vi "TestExec.Test Metric Add_Get.vi"(7 "Log Dir":path=path "C:/MTE/Circle Test/Logs", 8 "Max Hist Len":i32=10000, 9 "Test Record":T2, 10 "Action":T1, 11 "Test Result Metrics":T5) -> (1 "Test History":T4, 3 "Test Result Metrics Out":T5)   [LabVIEW 2018]
uses:
  TestExec.Test Result Metric Status.ctl
  TestExec.Test Result Metric History.ctl
  TestExec.Test Result Metric History Item.ctl
  <vilib>/KATE/SeqMgr/SeqMgr.Result State Enum.ctl
  TestExec.Test Metric Action Selector.ctl
  <vilib>/KATE/Files/File Utils.lvlib
  <vilib>/KATE/SeqMgr/SeqMgr.lvlib
panel:
  # "Time                                           Test/UUT                      Result/Code                                 Description"
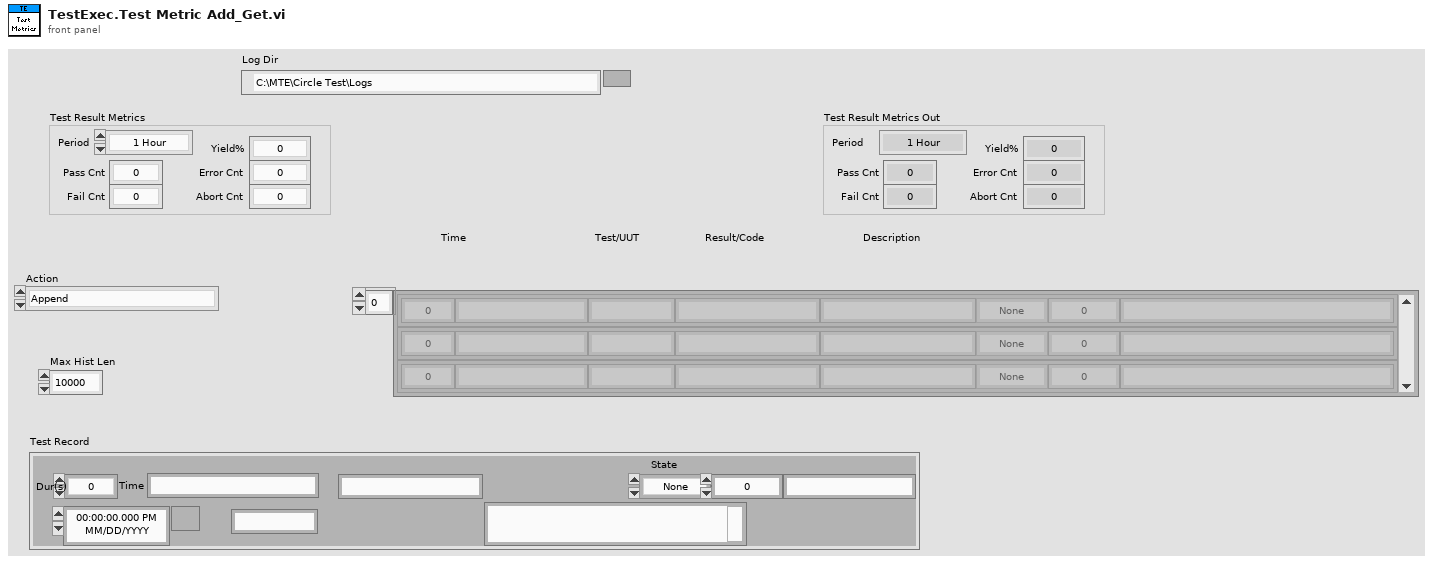
[diagram p1: front panel]
types:
  T1 = typedef "TestExec.Test Metric Action Selector.ctl" = enum16{"Append", "Get Metrics", "Reset", "Load", "Save"}
  T2 = typedef "TestExec.Test Result Metric History Item.ctl" = cluster{"TimeStamp":timestamp, "Dur(s)":dbl, "Time":string, "Mode ":string, "Test ":string, "SN":string, "State":T3, "Code":i32, "Description":string}
  T3 = typedef "KATE_Lib.lvlib/SeqMgr.lvlib/SeqMgr.Result State Enum.ctl" = enum16{"None", "Passing", "Failing", "PASS", "FAIL", "ABORT", "ERROR"}
  T4 = typedef "TestExec.Test Result Metric History.ctl" = T2[]
  T5 = typedef "TestExec.Test Result Metric Status.ctl" = cluster{"Period":enum16{"1 Hour", "4 Hours", "1 Day", "1 Week"}, "Pass Cnt":i32, "Fail Cnt":i32, "Yield%":dbl, "Error Cnt":i32, "Abort Cnt":i32}
  T6 = enum16{"open", "replace", "create", "open or create", "replace or create", "replace or create with confirmation"}
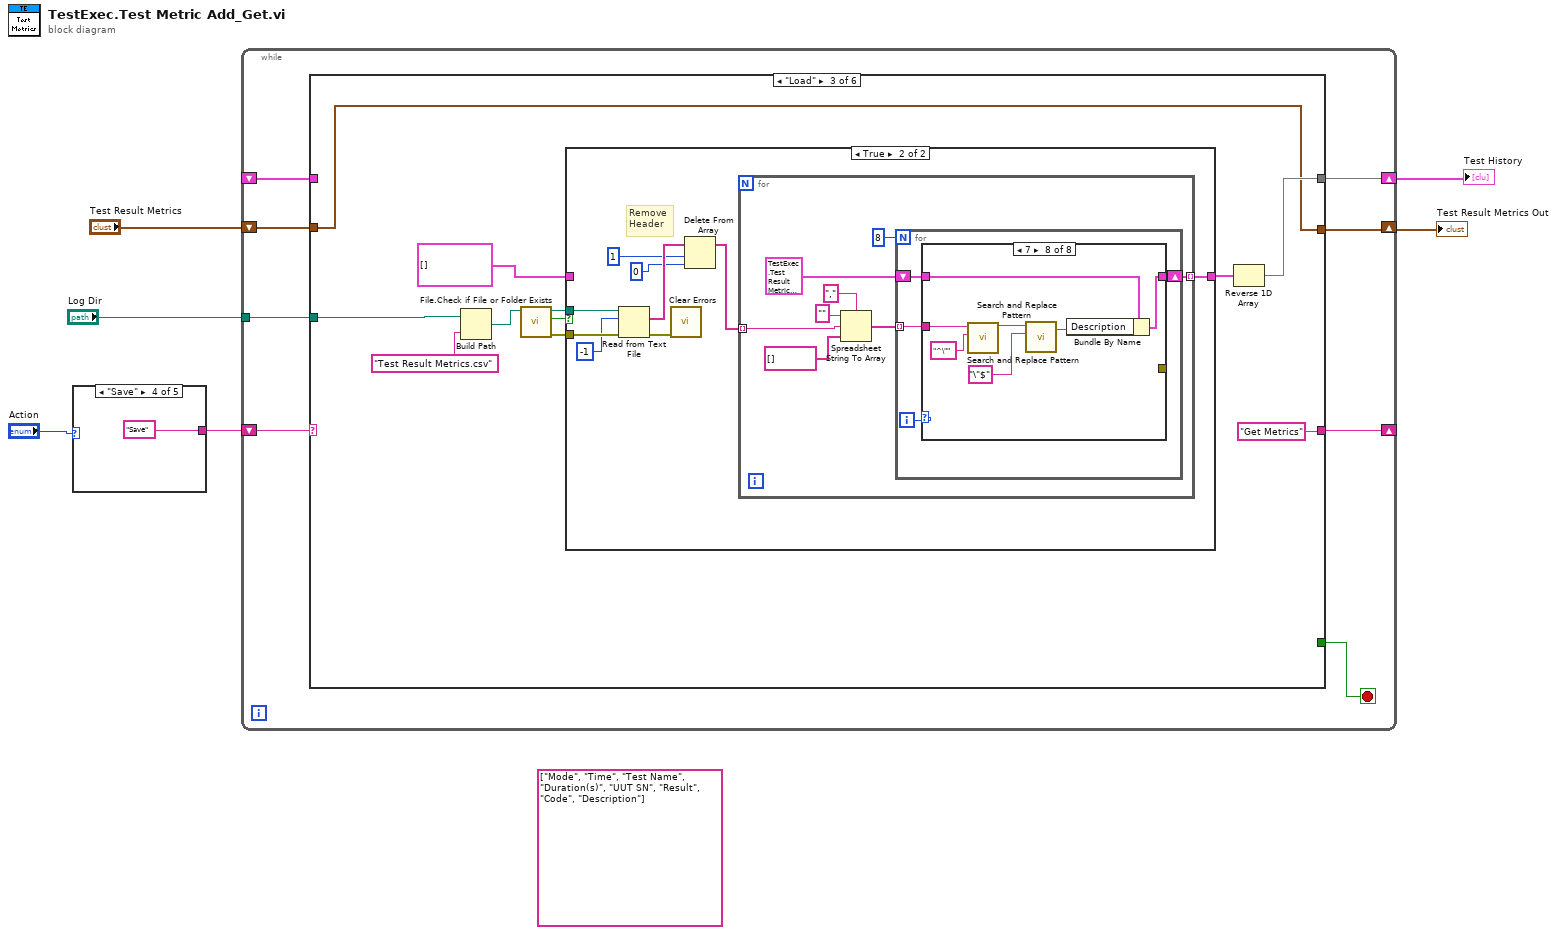
[diagram p0: block diagram]
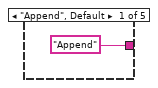
[diagram p2: hidden frame]
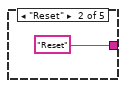
[diagram p3: hidden frame]
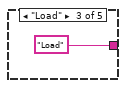
[diagram p4: hidden frame]
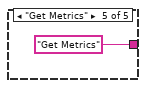
[diagram p5: hidden frame]
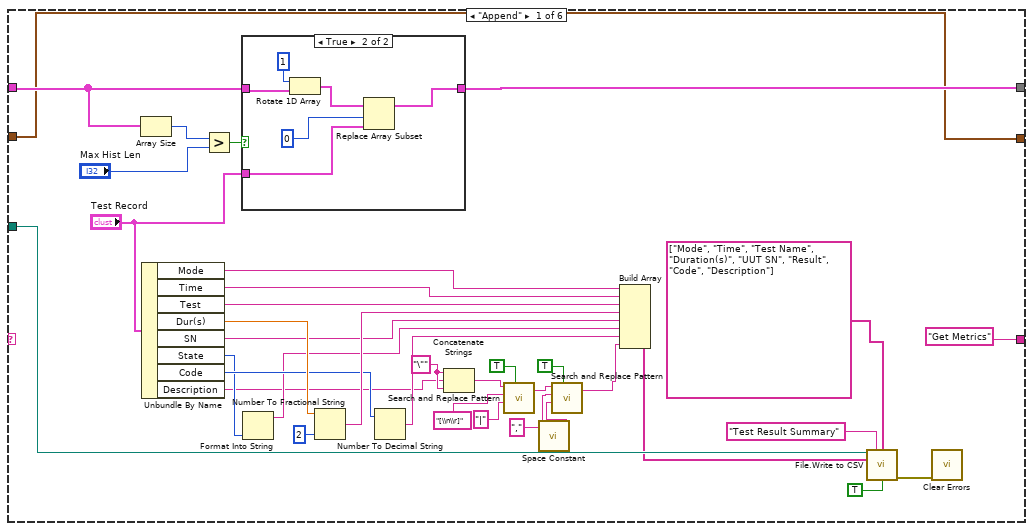
[diagram p6: hidden frame]
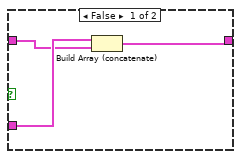
[diagram p7: hidden frame]
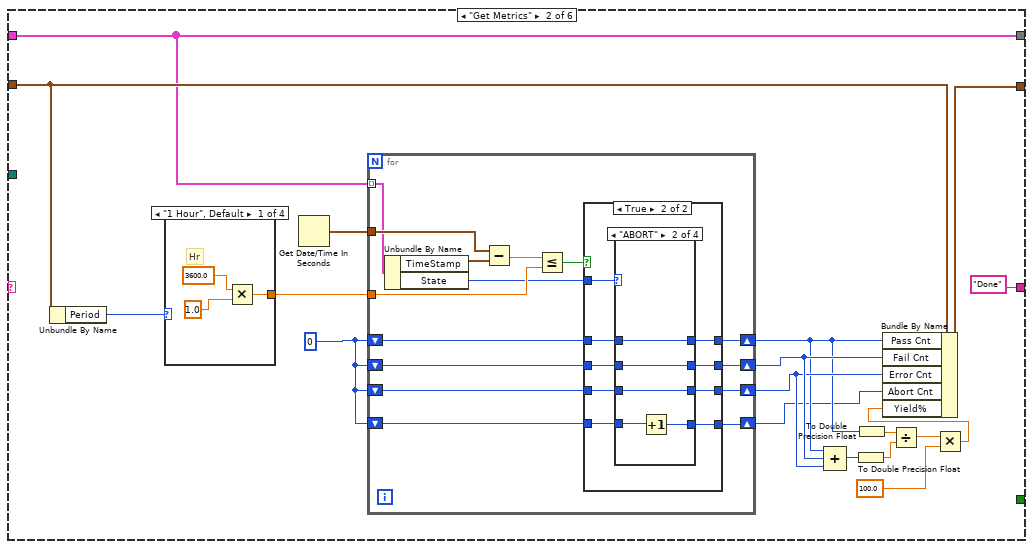
[diagram p8: hidden frame]
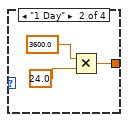
[diagram p9: hidden frame]
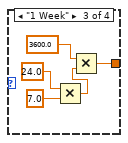
[diagram p10: hidden frame]
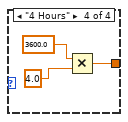
[diagram p11: hidden frame]
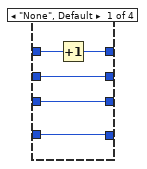
[diagram p13: hidden frame]
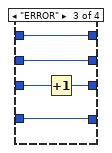
[diagram p14: hidden frame]
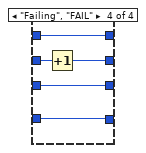
[diagram p15: hidden frame]
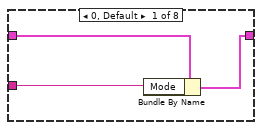
[diagram p17: hidden frame]
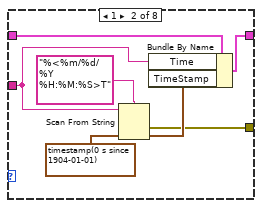
[diagram p18: hidden frame]
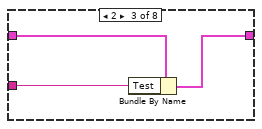
[diagram p19: hidden frame]
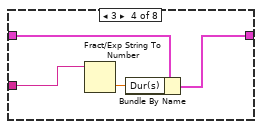
[diagram p20: hidden frame]
diagram:
  (unwired) string[] ["Mode", "Time", "Test Name", "Duration(s)", "UUT SN", "Result", "Code", "Description"] ("Header")
  n1 = case shown="\"Save\"" "Action" {
    tunnel: ["Append" "Reset" "Load" "Save" "Get Metrics"] -> w1
    frame "Append", Default {
    }
    frame "Reset" {
    }
    frame "Load" {
    }
    frame "Save" {
    }
    frame "Get Metrics" {
    }
  }
  n2 = while {
    shift-right: [w18] -> _
    shift-left: w1 -> [w19]
    shift-right: [w16] -> w4
    shift-left: _ -> [w15]
    tunnel: "Log Dir" -> [w12]
    shift-right: [w14] -> w5
    shift-left: "Test Result Metrics" -> [w17]
    stop <- w13 stop-if-true
    n3 = case shown="\"Load\"" w19 {
      tunnel: ["Get Metrics" "Done" "Get Metrics" "Get Metrics" "Done" "Done"] -> w18
      tunnel: w17 -> [w22 w79 w145 w215 w236 w264]
      tunnel: [w50 w69 w146 _ w217 w265] -> w16
      tunnel: w15 -> [w51 w69 _ _ w217 w265]
      tunnel: [w22 w70 w145 w215 w236 w264] -> w14
      tunnel: [_ _ _ _ _ TRUE] -> w13
      tunnel: w12 -> [w46 _ w148 _ w222 _]
      frame "Append" {
        w34 = "\""
        n4 = Array Size(array=w51) -> (size(s)=w54:i32)
        n5 = Unbundle By Name("Test Record") -> ("Mode"=w20:string, "Time"=w23:string, "Test"=w45:string, "Dur(s)"=w44:dbl, "SN"=w41:string, "State"=w38:T3, "Code"=w40:i32, "Description"=w33:string)
        n6 = Greater?(x=w54, y="Max Hist Len") -> (0:w52:bool)
        n7 = case shown="True" w52 {
          tunnel: w51 -> [w56 w61]
          tunnel: [w58 w60] -> w50
          tunnel: "Test Record" -> [w57 w59]
          frame False {
            n8 = Build Array (concatenate)(w57, w56) -> (w58:T2[])
          }
          frame True {
            n9 = Rotate 1D Array(1:w61, 2:1 ("index")) -> (0:w64:T2[])
            n10 = Replace Array Subset(array=w64, new element=w59, index=0) -> (w60:T2[])
          }
        }
        n11 = Format Into String(w38) -> (resulting string=w37:string)  [unwired: 3 in, 1 out]
        n12 = Number To Fractional String(number=w44, precision (6)=i16 2) -> (F-format string=w42:string)  [unwired: 2 in]
        n13 = Number To Decimal String(number=w40) -> (decimal integer string=w39:string)  [unwired: 1 in]
        n14 = Concatenate Strings(w34, w33, w34) -> (w32:string)
        n15 = call <vilib>:"Search and Replace Pattern.vi"("string"=w32, "regular expression (\"\")"="[\\n\\r]", "replace string (\"\")"="|", "replace all? (F)"=TRUE) -> ("result string"=w28:string)  [unwired: 1 in, 1 out]
        n16 = call <vilib>:"Space Constant.vi"() -> ("String"=w25:string)
        n17 = call <vilib>:"Search and Replace Pattern.vi"("string"=w28, "regular expression (\"\")"=",", "replace string (\"\")"=w25, "replace all? (F)"=TRUE) -> ("result string"=w24:string)  [unwired: 1 in, 1 out]
        n18 = Build Array(w20, w23, w45, w42, w41, w37, w39, w24) -> (w35:string[])
        n19 = call <vilib>:"File.Write to CSV.vi"("Folder"=w46, "FileRootName"="Test Result Summary", "Header"=string[] ["Mode", "Time", "Test Name", "Duration(s)", "UUT SN", "Result", "Code", "Description"], "1D"=w35, "Append Date to Filename"=TRUE) -> ("error out"=w48:errorcluster)  [unwired: 9 in, 1 out]
        n20 = call <vilib>:"Clear Errors.vi"("error in (no error)"=w48) -> ()  [unwired: 5 in, 2 out]
      }
      frame "Get Metrics" {
        w67 = 0
        n21 = Unbundle By Name(w79) -> ("Period"=w81:enum16{"1 Hour", "4 Hours", "1 Day", "1 Week"})
        n22 = case shown="\"1 Hour\", Default" w81 {
          tunnel: [w83 w86 w92 w94] -> w80
          frame "1 Hour", Default {
            # "Hr"
            n23 = Multiply(x=3600.0, y=1.0) -> (x*y=w83:dbl)
          }
          frame "1 Day" {
            n24 = Multiply(x=3600.0, y=24.0) -> (x*y=w86:dbl)
          }
          frame "1 Week" {
            n25 = Multiply(x=24.0, y=7.0) -> (x*y=w89:dbl)
            n26 = Multiply(x=3600.0, y=w89) -> (x*y=w92:dbl)
          }
          frame "4 Hours" {
            n27 = Multiply(x=3600.0, y=4.0) -> (x*y=w94:dbl)
          }
        }
        n28 = Get Date/Time In Seconds() -> (seconds since 1Jan1904=w68:timestamp)
        n29 = for {
          tunnel: w69 -> [w100] mode=indexing
          tunnel: w68 -> [w110]
          tunnel: w80 -> [w108]
          shift-right: [w105] -> w74
          shift-left: w67 -> [w106]
          shift-right: [w103] -> w78
          shift-left: w67 -> [w104]
          shift-right: [w101] -> w77
          shift-left: w67 -> [w102]
          shift-right: [w97] -> w65
          shift-left: w67 -> [w98]
          n30 = Unbundle By Name(w100) -> ("TimeStamp"=w111:timestamp, "State"=w107:T3)
          n31 = Subtract(x=w110, y=w111) -> (x-y=w109:dbl)
          n32 = Less Or Equal?(x=w109, y=w108) -> (x <= y?=w99:bool)
          n33 = case shown="True" w99 {
            tunnel: w107 -> [_ w124]
            tunnel: w106 -> [w115 w123]
            tunnel: [w115 w122] -> w105
            tunnel: w104 -> [w114 w121]
            tunnel: [w114 w120] -> w103
            tunnel: w102 -> [w113 w119]
            tunnel: [w113 w118] -> w101
            tunnel: w98 -> [w112 w117]
            tunnel: [w112 w116] -> w97
            frame False {
            }
            frame True {
              n34 = case shown="\"ABORT\"" w124 {
                tunnel: w123 -> [w129 w134 w139 w144]
                tunnel: [w128 w134 w139 w144] -> w122
                tunnel: w121 -> [w127 w133 w138 w143]
                tunnel: [w127 w133 w138 w142] -> w120
                tunnel: w119 -> [w126 w130 w137 w141]
                tunnel: [w126 w130 w136 w141] -> w118
                tunnel: w117 -> [w125 w132 w135 w140]
                tunnel: [w125 w131 w135 w140] -> w116
                frame "None", Default {
                  n35 = Increment(x=w129) -> (x+1=w128:i32)
                }
                frame "ABORT" {
                  n36 = Increment(x=w132) -> (x+1=w131:i32)
                }
                frame "ERROR" {
                  n37 = Increment(x=w137) -> (x+1=w136:i32)
                }
                frame "Failing", "FAIL" {
                  n38 = Increment(x=w143) -> (x+1=w142:i32)
                }
              }
            }
          }
        }
        n39 = Compound Arithmetic op=ADD(w74, w78, w77) -> (w76:i32)
        n40 = To Double Precision Float(number=w76) -> (double precision float=w75:dbl)
        n41 = To Double Precision Float(number=w74) -> (double precision float=w73:dbl)
        n42 = Divide(x=w73, y=w75) -> (x/y=w72:dbl)
        n43 = Multiply(x=w72, y=100.0) -> (x*y=w66:dbl)
        n44 = Bundle By Name(cluster=w79, "Pass Cnt"=w74, "Fail Cnt"=w78, "Error Cnt"=w77, "Abort Cnt"=w65, "Yield%"=w66) -> (w70:T5)
      }
      frame "Load" {
        n45 = Build Path(base path=w148, name or relative path="Test Result Metrics.csv") -> (appended path=w154:path)
        n46 = call <vilib>:"File.Check if File or Folder Exists.vi"("Path"=w154) -> ("error out"=w152:errorcluster, "Exists"=w153:bool, "Dup Path"=w151:path)  [unwired: 6 in, 2 out]
        n47 = case shown="True" w153 {
          tunnel: w152 -> [_ w164]
          tunnel: w151 -> [_ w165]
          tunnel: [w156 w161] -> w147
          tunnel: T2[] [] -> [w156 _]
          frame False {
          }
          frame True {
            # "Remove\nHeader"
            n48 = Read from Text File(file (use dialog)=w165, count=-1, error in=w164) -> (text=w160:string[], error out=w162:errorcluster)  [unwired: 1 in, 2 out]
            n49 = call <vilib>:"Clear Errors.vi"("error in (no error)"=w162) -> ()  [unwired: 5 in, 2 out]
            n50 = Delete From Array(array=w160, length=1, index=0 ("length")) -> (array with subset deleted=w157:string[])  [unwired: 1 out]
            n51 = for {
              tunnel: w157 -> [w170] mode=indexing
              tunnel: [w166] -> w161 mode=indexing
              n52 = Spreadsheet String To Array(delimiter (Tab)=",", format string="", spreadsheet string=w170, array type (2D Dbl)=string[] []) -> (array=w169:string[])
              n53 = for {
                N: 8 -> [_]
                tunnel: w169 -> [w174] mode=indexing
                shift-right: [w175] -> w166
                shift-left: T2 {"TimeStamp"=timestamp(0 s since 1904-01-01), "Dur(s)"=0.0, "Time"="", "Mode "="", "Test "="", "SN"="", "State"=enum."None", "Code"=0, "Description"=""} ("Test Record") -> [w176]
                i -> [w177]
                n54 = case shown="7" w177 {
                  tunnel: w176 -> [w180 w187 w190 w194 w197 w203 w207 w214]
                  tunnel: [w179 w186 w189 w193 w196 w202 w206 w213] -> w175
                  tunnel: w174 -> [w178 w182 w188 w192 w195 w200 w205 w212]
                  tunnel: [_ w181 _ _ _ _ _ _] -> _
                  frame 0, Default {
                    n55 = Bundle By Name(cluster=w180, "Mode"=w178) -> (w179:T2)
                  }
                  frame 1 {
                    n56 = Scan From String(format string="%<%m/%d/%Y %H:%M:%S>T", input string=w182, default 1=timestamp(0 s since 1904-01-01)) -> (error out=w181:errorcluster, output 1=w183:timestamp)  [unwired: 2 in, 2 out]
                    n57 = Bundle By Name(cluster=w187, "Time"=w182, "TimeStamp"=w183) -> (w186:T2)
                  }
                  frame 2 {
                    n58 = Bundle By Name(cluster=w190, "Test"=w188) -> (w189:T2)
                  }
                  frame 3 {
                    n59 = Fract/Exp String To Number(string=w192) -> (number=w191:dbl)  [unwired: 3 in, 1 out]
                    n60 = Bundle By Name(cluster=w194, "Dur(s)"=w191) -> (w193:T2)
                  }
                  frame 4 {
                    n61 = Bundle By Name(cluster=w197, "SN"=w195) -> (w196:T2)
                  }
                  frame 5 {
                    n62 = Scan From String(format string="%s", input string=w200, default 1=SeqMgr.Result_State_Enum."None" ("State")) -> (output 1=w201:T3)  [unwired: 2 in, 3 out]
                    n63 = Bundle By Name(cluster=w203, "State"=w201) -> (w202:T2)
                  }
                  frame 6 {
                    n64 = Decimal String To Number(string=w205) -> (number=w204:i32)  [unwired: 2 in, 1 out]
                    n65 = Bundle By Name(cluster=w207, "Code"=w204) -> (w206:T2)
                  }
                  frame 7 {
                    n66 = call <vilib>:"Search and Replace Pattern.vi"("string"=w212, "regular expression (\"\")"="^\"") -> ("result string"=w210:string)  [unwired: 3 in, 1 out]
                    n67 = call <vilib>:"Search and Replace Pattern.vi"("string"=w210, "regular expression (\"\")"="\"$") -> ("result string"=w209:string)  [unwired: 3 in, 1 out]
                    n68 = Bundle By Name(cluster=w214, "Description"=w209) -> (w213:T2)
                  }
                }
              }
            }
          }
        }
        n69 = Reverse 1D Array(array=w147) -> (reversed array=w146:T2[])
      }
      frame "Reset" {
      }
      frame "Save" {
        n70 = Reverse 1D Array(array=w217) -> (reversed array=w218:T2[])
        n71 = for {
          tunnel: [w254] -> w219 mode=indexing
          tunnel: w218 -> [w253] mode=indexing
          w250 = "\""
          n72 = Unbundle By Name(w253) -> ("Mode"=w238:string, "Time"=w239:string, "Test"=w261:string, "Dur(s)"=w260:dbl, "SN"=w257:string, "State"=w252:T3, "Code"=w256:i32, "Description"=w241:string)
          n73 = Format Into String(w252) -> (resulting string=w251:string)  [unwired: 3 in, 1 out]
          n74 = Number To Fractional String(number=w260, precision (6)=i16 2) -> (F-format string=w258:string)  [unwired: 2 in]
          n75 = Number To Decimal String(number=w256) -> (decimal integer string=w255:string)  [unwired: 1 in]
          n76 = Concatenate Strings(w250, w241, w250) -> (w249:string)
          n77 = call <vilib>:"Search and Replace Pattern.vi"("string"=w249, "regular expression (\"\")"="[\\n\\r]", "replace string (\"\")"="|", "replace all? (F)"=TRUE) -> ("result string"=w245:string)  [unwired: 1 in, 1 out]
          n78 = call <vilib>:"Space Constant.vi"() -> ("String"=w242:string)
          n79 = call <vilib>:"Search and Replace Pattern.vi"("string"=w245, "regular expression (\"\")"=",", "replace string (\"\")"=w242, "replace all? (F)"=TRUE) -> ("result string"=w240:string)  [unwired: 1 in, 1 out]
          n80 = Build Array(w238, w239, w261, w258, w257, w251, w255, w240) -> (w254:string[])
        }
        n81 = call <vilib>:"File.Create Folder if Does Not Exist.vi"("Path"=w222) -> ("error out"=w220:errorcluster, "Dup Path"=w221:path)  [unwired: 8 in, 1 out]
        n82 = Build Path(base path=w221, name or relative path="Test Result Metrics.csv") -> (appended path=w223:path)
        n83 = Open/Create/Replace File(file path (use dialog)=w223, error in=w220, operation (0:open)=T6."replace or create") -> (refnum out=w230:refnum<file>, error out=w231:errorcluster)  [unwired: 3 in, 1 out]
        n84 = Build Array (concatenate)(string[] ["Mode", "Time", "Test Name", "Duration(s)", "UUT SN", "Result", "Code", "Description"] ("Header"), w219) -> (w226:string[][])
        n85 = Array To Spreadsheet String(delimiter (Tab)=",", array=w226, 3:"" ("format string")) -> (spreadsheet string=w225:string)
        n86 = Write to Text File(file (use dialog)=w230, text=w225, error in=w231) -> (refnum out=w233:refnum<file>, error out=w234:errorcluster)  [unwired: 1 in, 1 out]
        n87 = Close File(refnum=w233, error in=w234) -> (error out=w224:errorcluster)  [unwired: 1 out]
        n88 = call <vilib>:"Clear Errors.vi"("error in (no error)"=w224) -> ()  [unwired: 5 in, 2 out]
      }
      frame "Done", Default {
      }
    }
  }
  "Test Result Metrics Out" <- w5
  "Test History" <- w4
